vi "Check Input String.vi"(5 "Drop-down List Options":string[](array[string]), 7 "Allow Undefined Strings":bool, 11 "String in":string) -> (3 "String out":string)   [LabVIEW 2018, in "List Data Type.lvclass"]
uses:
  List Data Type.lvclass
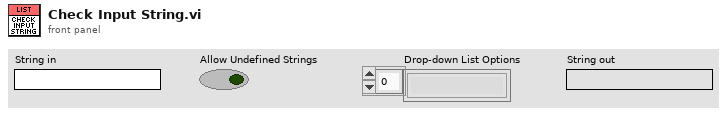
[diagram p1: front panel]
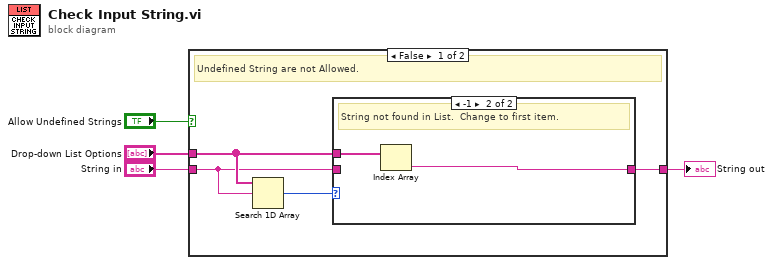
[diagram p0: block diagram]
diagram:
  n1 = case shown="False" "Allow Undefined Strings" {
    tunnel: "String in" -> [w5 w12]
    tunnel: [w6 w12] -> w2
    tunnel: "Drop-down List Options" -> [w7 _]
    frame False {
      # "Undefined String are not Allowed."
      n2 = Search 1D Array(1D array=w7, element=w5) -> (index of element=w8:i32)  [unwired: 1 in]
      n3 = case shown="-1" w8 {
        tunnel: w7 -> [_ w11]
        tunnel: [w9 w10] -> w6
        tunnel: w5 -> [w9 _]
        frame Default {
          # "String found in list.  Accept input."
        }
        frame -1 {
          # "String not found in List.  Change to first item."
          n4 = Index Array(array=w11) -> (element=w10:string)  [unwired: 1 in]
        }
      }
    }
    frame True {
      # "Undefined Strings are Allowed.  Accept any input."
    }
  }
  "String out" <- w2
